vi "Global-TestcaseCSM.vi"() -> ()   [LabVIEW 2017, in "CSM-Testcase.lvlib"]
uses:
  CSM-Testcase.lvlib
panel:
  in  "response":T1
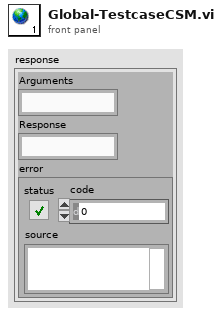
[diagram p1: front panel]
types:
  T1 = cluster{"Arguments":string, "Response":string, "error":errorcluster}
diagram:
